vi "Liquid Lens serial input.vi"(8 "错误输入（无错误）":errorcluster, 9 "parameter":u16, 10 "item":u8, 11 "VISA资源名称":refnum<visa-resource-name>) -> (0 "错误输出":errorcluster, 3 "VISA资源名称输出":refnum<visa-resource-name>)   [LabVIEW 2015, in "Serial.lvlib"]
uses:
  Serial.lvlib
panel:
  # "item为写入属性，1为转速，2为正传，3为反转。\nparameter为写入参数，属性为转速时，则写入\n转速大小，如1000为1000Hz，最大转速为2000Hz，\n当设置转速大于2000时，则下位机设置为2000Hz。\n当属性为2或者3时，设置的参数为脉冲产生的时间，\n单位mm，如1000则为1000mm里面输出脉冲信号。"
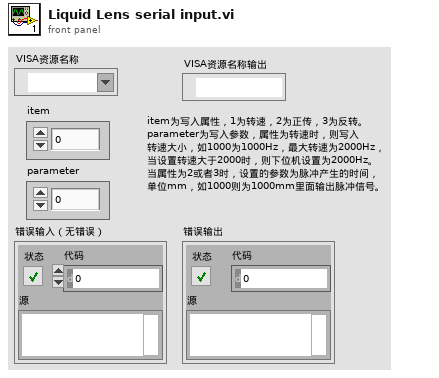
[diagram p1: front panel]
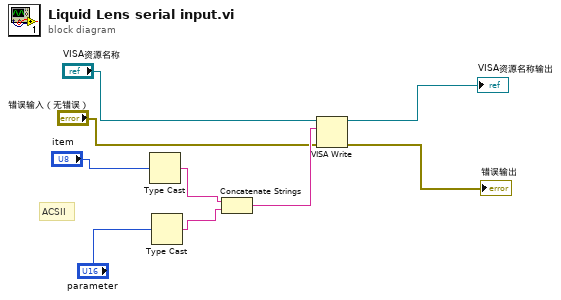
[diagram p0: block diagram]
diagram:
  # "ACSII"
  n1 = Type Cast(x="item") -> (*(type *) &x=w8:string)  [unwired: 1 in]
  n2 = Type Cast(x="parameter") -> (*(type *) &x=w7:string)  [unwired: 1 in]
  n3 = Concatenate Strings(w8, w7) -> (w6:string)
  n4 = VISA Write(VISA resource name="VISA资源名称", write buffer=w6, error in (no error)="错误输入（无错误）") -> (VISA resource name out=→"VISA资源名称输出":refnum<visa-resource-name>, error out=→"错误输出":errorcluster)  [unwired: 1 out]
